vi "Initialize Device Core.vi"(8 "error in (no error)":errorcluster, 9 "Reset (F)":bool, 10 "Resource Name":string, 11 "LS218 in":refnum<class "LS218.lvclass">) -> (0 "error out":errorcluster, 3 "LS218 out":refnum<class "LS218.lvclass">)   [LabVIEW 2013, in "LS218.lvlib" / "LS218.lvclass"]
doc: "Initialize device driver."
uses:
  LS218.lvclass
  CSPP_Core/Actors/CS++DeviceActor/CS++DeviceActor.lvclass
  CSPP_Core/Actors/CS++DeviceActor/CS++DeviceActor.lvclass/CS++DeviceActor.ctl
  LS218.lvclass/LS218.ctl
  CSPP_Core/Actors/CS++DeviceActor/Read ResetWithDefaults.vi
  <instrlib>/Lake Shore Cryotronics 218/Lake Shore Cryotronics 218.lvlib
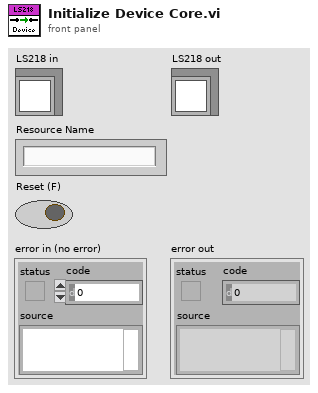
[diagram p1: front panel]
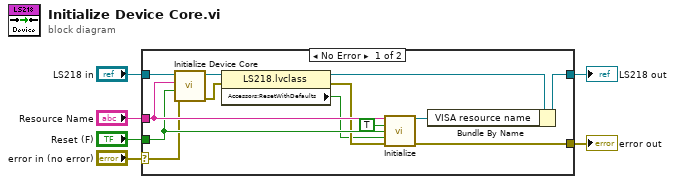
[diagram p0: block diagram]
diagram:
  n1 = case shown="No Error" "error in (no error)" {
    selector: "error in (no error)" -> [w12 w20]
    tunnel: "LS218 in" -> [w19 w21]
    tunnel: "Resource Name" -> [w18 _]
    tunnel: "Reset (F)" -> [w17 _]
    tunnel: [w14 w21] -> w3
    tunnel: [w13 w20] -> w2
    frame No Error {
      n2 = call-parent "Initialize Device Core.vi"("error in (no error)"=w12, "Reset (F)"=w17, "Resource Name"=w18, "CS++DeviceActor in"=w19) -> ("error out"=w9:errorcluster, "CS++DeviceActor out"=w11:refnum<class "LS218.lvclass">)  [unwired: 6 in]
      n3 = property class="LS218.lvclass"(reference=w11, error in=w9) -> (reference out=w10:refnum<class "LS218.lvclass">, error out=w8:errorcluster, "Accessors:ResetWithDefaults"=w7:bool)
      n4 = call <instrlib>:"Initialize.vi"("VISA resource name"=w18, "ID Query (T: Check)"=TRUE, "Reset (T: Reset)"=w17, "Reset Defaults (F:Dont Reset)"=w7, "error in (no error)"=w8) -> ("VISA resource name out"=w15:refnum<visa-resource-name>, "error out"=w13:errorcluster)  [unwired: 9 in]
      n5 = Bundle By Name(cluster=w10, "VISA resource name"=w15) -> (w14:refnum<class "LS218.lvclass">)
    }
    frame Error {
    }
  }
  "error out" <- w2
  "LS218 out" <- w3
